vi "Write TDMS.vi"(8 "error in (no error)":errorcluster, 9 "Timed out? (False)":bool, 10 "Distance (m)":dbl, 11 "Devantech SRF05 in":refnum<class "Devantech SRF05.lvclass">) -> (0 "error out":errorcluster, 3 "Devantech SRF05 out":refnum<class "Devantech SRF05.lvclass">)   [LabVIEW 2019, in "Devantech SRF05.lvclass"]
doc: "Writes data to the tdms file. Call Open TDMS VI before running this VI."
uses:
  Devantech SRF05.lvclass
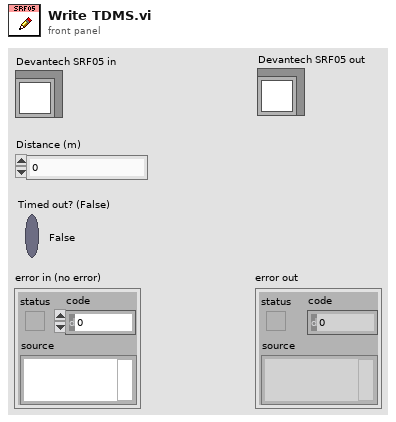
[diagram p1: front panel]
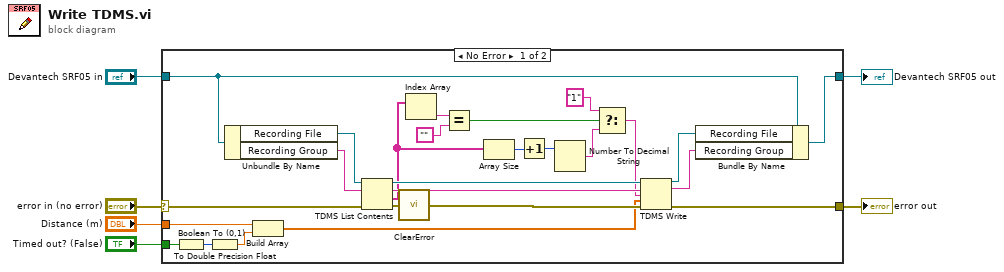
[diagram p0: block diagram]
diagram:
  n1 = case shown="No Error" "error in (no error)" {
    selector: "error in (no error)" -> [w25 w34]
    tunnel: [w32 w34] -> w4
    tunnel: [w28 w33] -> w3
    tunnel: "Devantech SRF05 in" -> [w31 w33]
    tunnel: "Distance (m)" -> [w11 _]
    tunnel: "Timed out? (False)" -> [w8 _]
    frame No Error {
      n2 = Boolean To (0,1)(Boolean=w8) -> (0, 1=w10:i16)
      n3 = To Double Precision Float(number=w10) -> (double precision float=w9:dbl)
      n4 = Unbundle By Name(w31) -> ("Recording File"=w27:refnum<k34>, "Recording Group"=w26:string)
      n5 = Build Array(w11, w9) -> (w12:dbl[])
      n6 = TDMS List Contents(4:w25, 6:w26, 7:w27) -> (0:w7:errorcluster, 1:w15:string[], 2:w24:string, 3:w23:refnum<k34>)
      n7 = call <vilib>:"ClearError.vi"("error in (no error)"=w7) -> ("error out"=w20:errorcluster)
      n8 = Index Array(array=w15) -> (element=w19:string)  [unwired: 1 in]
      n9 = Equal?(x=w19, y="") -> (x = y?=w17:bool)
      n10 = Array Size(array=w15) -> (size(s)=w22:i32)
      n11 = Increment(x=w22) -> (x+1=w21:i32)
      n12 = Number To Decimal String(number=w21) -> (decimal integer string=w14:string)  [unwired: 1 in]
      n13 = Select(t="1", s=w17, f=w14) -> (s? t:f=w13:string)
      n14 = TDMS Write(0:w23, 5:w24, 7:w13, 9:w12, 11:w20) -> (4:w30:refnum<k34>, 6:w29:string, 15:w32:errorcluster)  [unwired: 1 in, 1 out]
      n15 = Bundle By Name(cluster=w31, "Recording File"=w30, "Recording Group"=w29) -> (w28:refnum<class "Devantech SRF05.lvclass">)
    }
    frame Error {
    }
  }
  "error out" <- w4
  "Devantech SRF05 out" <- w3
